vi "Process_NS3_Data.vi"(11 "Sim_results":string) -> (3 "Data":dbl[][](array[numeric]))   [LabVIEW 2010]
doc: "This VI implements the routine for translatings the NS3 simulation data into an array of values that can be processed later.\n\nCreated by Davis Montenegro\n06-28-2017"
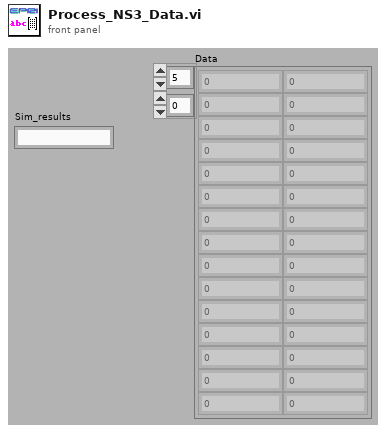
[diagram p1: front panel]
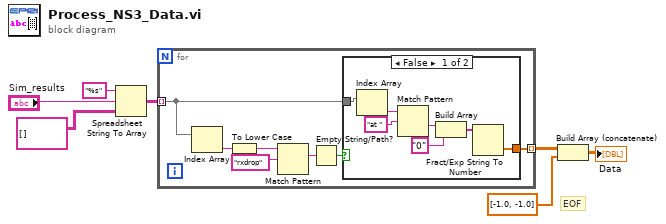
[diagram p0: block diagram]
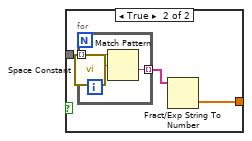
[diagram p2: hidden frame]
diagram:
  # "EOF"
  n1 = Spreadsheet String To Array(format string="%s", spreadsheet string="Sim_results", array type (2D Dbl)=string[][] []) -> (array=w4:string[][])  [unwired: 1 in]
  n2 = for {
    tunnel: w4 -> [w9] mode=indexing
    tunnel: [w8] -> w3 mode=indexing
    n3 = Index Array(array=w9) -> (element=w14:string)  [unwired: 1 in]
    n4 = To Lower Case(string=w14) -> (all lower case string=w13:string)
    n5 = Match Pattern(string=w13, regular expression="rxdrop") -> (match substring=w11:string)  [unwired: 1 in, 3 out]
    n6 = Empty String/Path?(string/path=w11) -> (empty?=w10:bool)
    n7 = case shown="False" w10 {
      tunnel: w9 -> [w21 w24]
      tunnel: [w15 w22] -> w8
      frame False {
        n8 = Index Array(array=w21) -> (element=w20:string)  [unwired: 1 in]
        n9 = Match Pattern(string=w20, regular expression="at ") -> (after substring=w18:string)  [unwired: 1 in, 3 out]
        n10 = Build Array(w18, "0") -> (w16:string[])
        n11 = Fract/Exp String To Number(string=w16) -> (number=w15:dbl[])  [unwired: 3 in, 1 out]
      }
      frame True {
        n12 = for {
          tunnel: w24 -> [w27] mode=indexing
          tunnel: [w25] -> w23 mode=indexing
          n13 = call <vilib>:"Space Constant.vi"() -> ("String"=w26:string)
          n14 = Match Pattern(string=w27, regular expression=w26) -> (after substring=w25:string)  [unwired: 1 in, 3 out]
        }
        n15 = Fract/Exp String To Number(string=w23) -> (number=w22:dbl[])  [unwired: 3 in, 1 out]
      }
    }
  }
  n16 = Build Array (concatenate)(w3, dbl[] [-1.0, -1.0]) -> (→"Data":dbl[][])
